vi "Read Collision state.vi"(11 "Collision in":refnum<class "Collision.lvclass">) -> (2 "Collision state":bool)   [LabVIEW 2021, in "Collision.lvclass"]
doc: "MIT Licence\nCopyright (c) 2024 David Grollier"
uses:
  Collision.lvclass
  Collision.lvclass/Collision.ctl
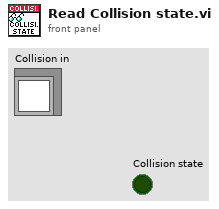
[diagram p1: front panel]
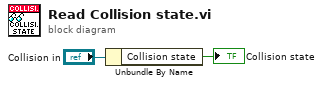
[diagram p0: block diagram]
diagram:
  n1 = Unbundle By Name("Collision in") -> ("Collision state"=→"Collision state":bool)
